vi "CalCanSigValue.vi"(8 "Col Index Map":map{string, i32}(c390), 9 "MeasData":dbl[](array[numeric]), 10 "RawData":u8[](array[numeric]), 11 "SignalFormat":T1) -> (3 "MeasData.out":dbl[](array[numeric]))   [LabVIEW 2024]
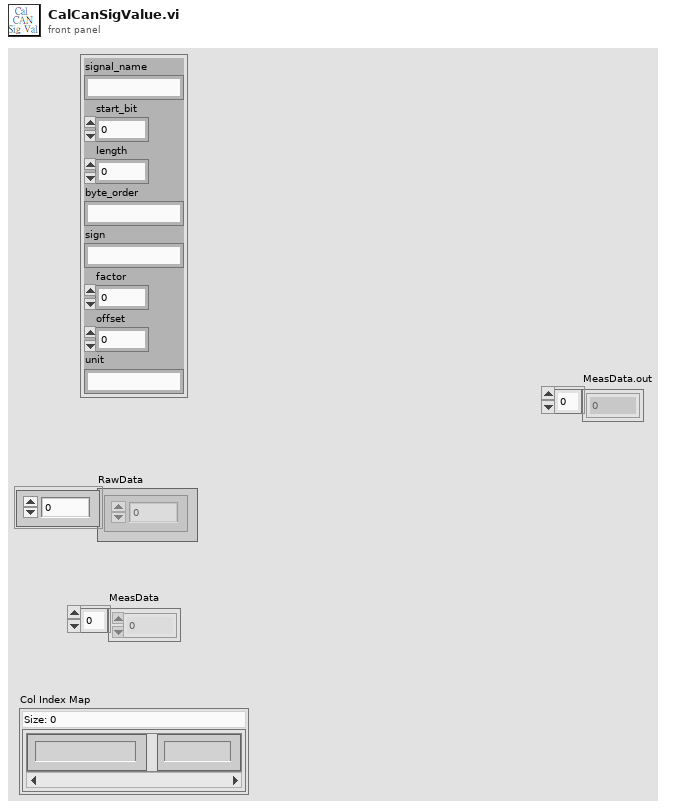
[diagram p1: front panel]
types:
  T1 = cluster{"signal_name":string, "start_bit":i32, "length":i32, "byte_order":string, "sign":string, "factor":dbl, "offset":dbl, "unit":string}
  T2 = enum16{"big-endian, network order", "native, host order", "little-endian"}
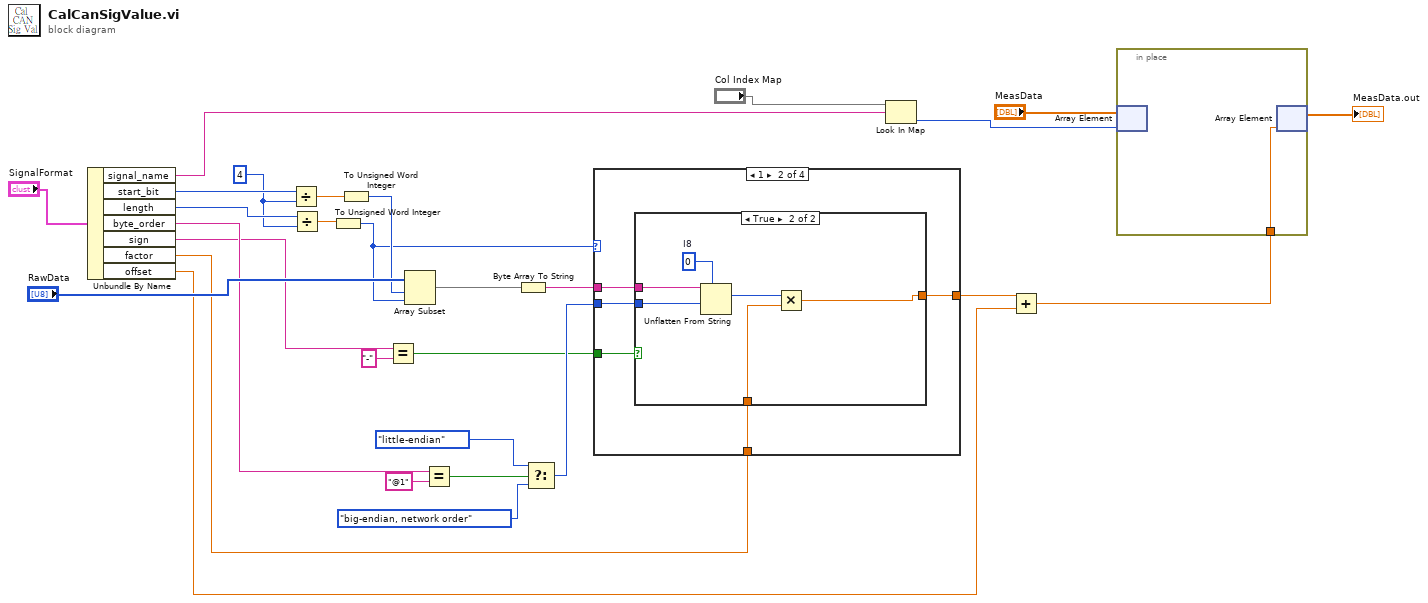
[diagram p0: block diagram]
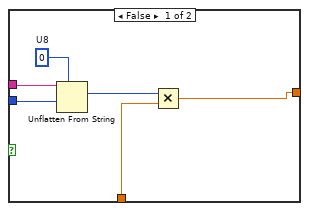
[diagram p3: hidden frame]
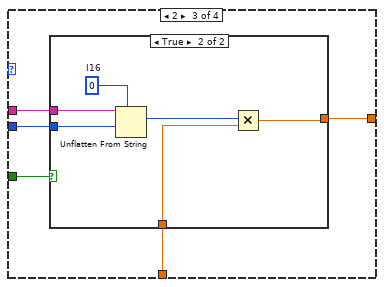
[diagram p4: hidden frame]
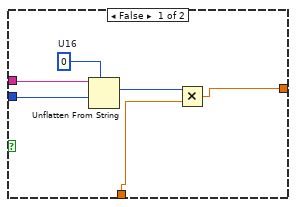
[diagram p5: hidden frame]
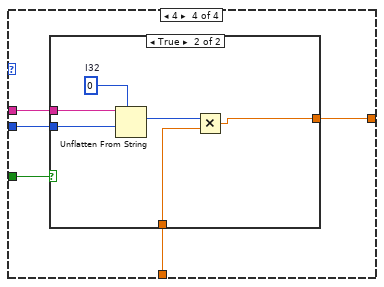
[diagram p6: hidden frame]
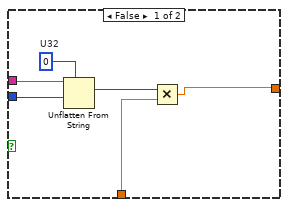
[diagram p7: hidden frame]
diagram:
  w26 = 4 ("y")
  n1 = Unbundle By Name("SignalFormat") -> ("signal_name"=w5:string, "start_bit"=w28:i32, "length"=w27:i32, "byte_order"=w21:string, "sign"=w19:string, "factor"=w8:dbl, "offset"=w11:dbl)
  n2 = Divide(x=w28, y=w26) -> (x/y=w24:dbl)
  n3 = Divide(x=w27, y=w26) -> (x/y=w23:dbl)
  n4 = To Unsigned Word Integer(number=w23) -> (unsigned 16bit integer=w10:u16)
  n5 = To Unsigned Word Integer(number=w24) -> (unsigned 16bit integer=w22:u16)
  n6 = Equal?(x=w19, y="-") -> (x = y?=w9:bool)
  n7 = Array Subset(array="RawData", index=w22, length=w10) -> (w17:u8[])
  n8 = Equal?(x=w21, y="@1") -> (x = y?=w15:bool)
  n9 = Byte Array To String(unsigned byte array=w17) -> (string=w16:string)
  n10 = Select(t=T2."little-endian" ("byte order (0:big-endian, network order)"), s=w15, f=T2."big-endian, network order" ("byte order (0:big-endian, network order)")) -> (s? t:f=w12:T2)
  n11 = case shown="1" w10 {
    tunnel: w16 -> [_ w34 w51 w68]
    tunnel: w12 -> [_ w33 w50 w67]
    tunnel: [_ w32 w49 w66] -> w7
    tunnel: w9 -> [_ w31 w48 w65]
    tunnel: w8 -> [_ w30 w47 w64]
    frame 0, Default {
    }
    frame 1 {
      n12 = case shown="True" w31 {
        tunnel: w34 -> [w40 w46]
        tunnel: w33 -> [w39 w45]
        tunnel: [w35 w41] -> w32
        tunnel: w30 -> [w37 w43]
        frame False {
          w38 = u8 0  # U8
          n13 = Unflatten From String(type=w38, binary string=w40, byte order (0:big-endian, network order)=w39) -> (value=w36:u8)  [unwired: 2 in, 2 out]
          n14 = Multiply(x=w36, y=w37) -> (x*y=w35:dbl)
        }
        frame True {
          w44 = i8 0  # I8
          n15 = Unflatten From String(type=w44, binary string=w46, byte order (0:big-endian, network order)=w45) -> (value=w42:i8)  [unwired: 2 in, 2 out]
          n16 = Multiply(x=w42, y=w43) -> (x*y=w41:dbl)
        }
      }
    }
    frame 2 {
      n17 = case shown="True" w48 {
        tunnel: w51 -> [w57 w63]
        tunnel: w50 -> [w56 w62]
        tunnel: [w52 w58] -> w49
        tunnel: w47 -> [w53 w59]
        frame False {
          w55 = u16 0  # U16
          n18 = Unflatten From String(type=w55, binary string=w57, byte order (0:big-endian, network order)=w56) -> (value=w54:u16)  [unwired: 2 in, 2 out]
          n19 = Multiply(x=w54, y=w53) -> (x*y=w52:dbl)
        }
        frame True {
          w61 = i16 0  # I16
          n20 = Unflatten From String(type=w61, binary string=w63, byte order (0:big-endian, network order)=w62) -> (value=w60:i16)  [unwired: 2 in, 2 out]
          n21 = Multiply(x=w60, y=w59) -> (x*y=w58:dbl)
        }
      }
    }
    frame 4 {
      n22 = case shown="True" w65 {
        tunnel: w68 -> [w74 w80]
        tunnel: w67 -> [w73 w79]
        tunnel: [w69 w75] -> w66
        tunnel: w64 -> [w70 w76]
        frame False {
          w72 = u32 0  # U32
          n23 = Unflatten From String(type=w72, binary string=w74, byte order (0:big-endian, network order)=w73) -> (value=w71:u32)  [unwired: 2 in, 2 out]
          n24 = Multiply(x=w71, y=w70) -> (x*y=w69:dbl)
        }
        frame True {
          w78 = 0  # I32
          n25 = Unflatten From String(type=w78, binary string=w80, byte order (0:big-endian, network order)=w79) -> (value=w77:i32)  [unwired: 2 in, 2 out]
          n26 = Multiply(x=w77, y=w76) -> (x*y=w75:dbl)
        }
      }
    }
  }
  n27 = Look In Map(map="Col Index Map", key=w5) -> (value=w3:i32)  [unwired: 1 in, 1 out]
  n28 = Add(x=w7, y=w11) -> (x+y=w2:dbl)
  n29 = in-place {
    in-place-border: w2 -> [w81]
    n30 = in-place-array #1("MeasData", w3) -> ()  [unwired: 1 out]
    n31 = in-place-array #1(w81) -> (→"MeasData.out":dbl[])  [unwired: 1 out]
  }
